vi "INTELLIFAUCET Temp Flow.vi"(7 "Temperature (T), Flow (F)":bool, 8 "error in (no error)":errorcluster, 10 "uA Output":i32, 11 "VISA Refnum in":refnum<visa-resource-name>) -> (0 "error out":errorcluster, 3 "VISA Refnum out":refnum<visa-resource-name>)   [LabVIEW 2023]
uses:
  MW100/Type Definitions/HEWH MW100 Channel Numbers.ctl
  Type Definitions/HEWH Normally Open Valve Control.ctl
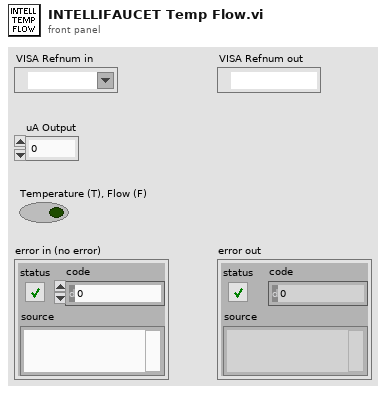
[diagram p1: front panel]
types:
  T1 = typedef "HEWH Normally Open Valve Control.ctl" = string
  T2 = typedef "HEWH MW100 Channel Numbers.ctl" = string
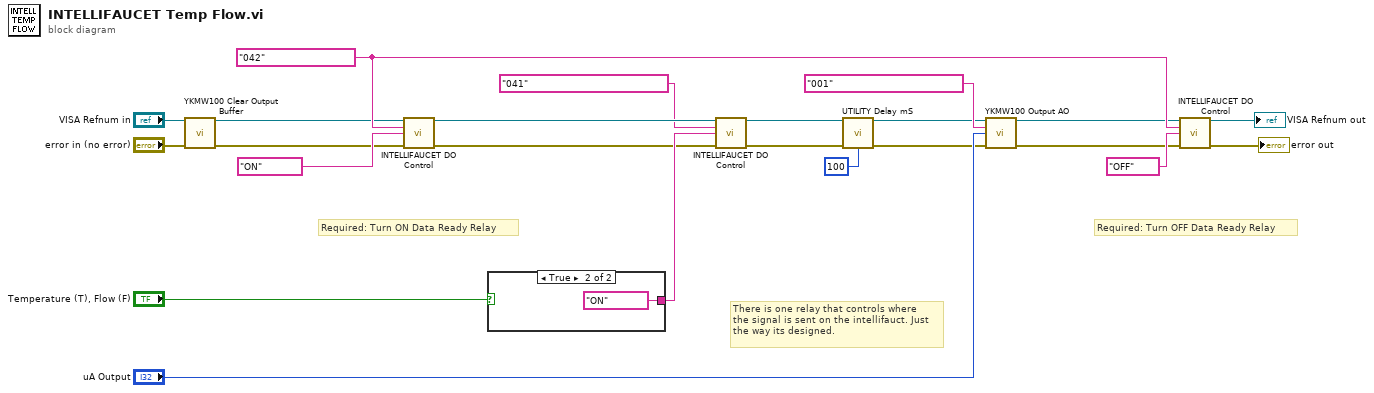
[diagram p0: block diagram]
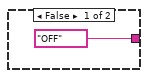
[diagram p2: hidden frame]
diagram:
  w19 = T2 "042" ("HEWH MW100 Channel Numbers")
  # "There is one relay that controls where\nthe signal is sent on the intellifauct. Just\nthe way its designed."
  # "Required: Turn OFF Data Ready Relay"
  # "Required: Turn ON Data Ready Relay"
  n1 = call "YKMW100 Clear Output Buffer.vi"("VISA session"="VISA Refnum in", "error in (no error)"="error in (no error)") -> ("dup VISA session"=w17:refnum<visa-resource-name>, "error out"=w16:errorcluster)  [unwired: 12 in]
  n2 = call "INTELLIFAUCET DO Control.vi"("VISA session"=w17, "HEWH MW100 Channel Numbers"=w19, "Normally Open"=T1 "ON" ("Normally Open Valve"), "Error In"=w16) -> ("dup VISA session"=w18:refnum<visa-resource-name>, "error out"=w1:errorcluster)  [unwired: 10 in]
  n3 = case shown="True" "Temperature (T), Flow (F)" {
    tunnel: [T1 "OFF" ("Normally Open Valve") T1 "ON" ("Normally Open Valve")] -> w8
    frame False {
    }
    frame True {
    }
  }
  n4 = call "INTELLIFAUCET DO Control.vi"("VISA session"=w18, "HEWH MW100 Channel Numbers"=T2 "041", "Normally Open"=w8, "Error In"=w1) -> ("dup VISA session"=w5:refnum<visa-resource-name>, "error out"=w3:errorcluster)  [unwired: 10 in]
  n5 = call "UTILITY Delay mS.vi"("Error In"=w3, "milliseconds to wait"=u32 100) -> ("Error Out"=w2:errorcluster)  [unwired: 13 in]
  n6 = call "YKMW100 Output AO.vi"("VISA session"=w5, "Channel String (001)"=T2 "001" ("HEWH MW100 Channel Numbers"), "Output Value (0)"="uA Output", "error in (no error)"=w2) -> ("dup VISA session"=w13:refnum<visa-resource-name>, "error out"=w12:errorcluster)  [unwired: 10 in]
  n7 = call "INTELLIFAUCET DO Control.vi"("VISA session"=w13, "HEWH MW100 Channel Numbers"=w19, "Normally Open"=T1 "OFF" ("Normally Open Valve"), "Error In"=w12) -> ("dup VISA session"=→"VISA Refnum out":refnum<visa-resource-name>, "error out"=→"error out":errorcluster)  [unwired: 10 in]
